vi "main - 截取字符显示.vi"() -> ()   [LabVIEW 2018]
uses:
  <vilib>/Instr/_visa.llb/VISA Configure Serial Port (Instr).vi
panel:
  out "波形图表 2":u32(graph)
  out "*(类型 *) &x 2":u32
  out "波形图表":u32(graph)
  out "Serial flag":bool
  out "*(类型 *) &x":u32
  out "子字符串 3":string
  out "子字符串 2":string
  out "子字符串":string
  out "枚举":T1
  out "返回数":u32
  in  "baud rate":u64(ring) items=["9600"=9600, "14400"=14400, "115200"=115200]
  out "read buffer":string
  out "serial_state":bool
  in  "serial":refnum<visa-resource-name> caption="serial_select"
  in  "serial_open":bool
  in  "exit":bool
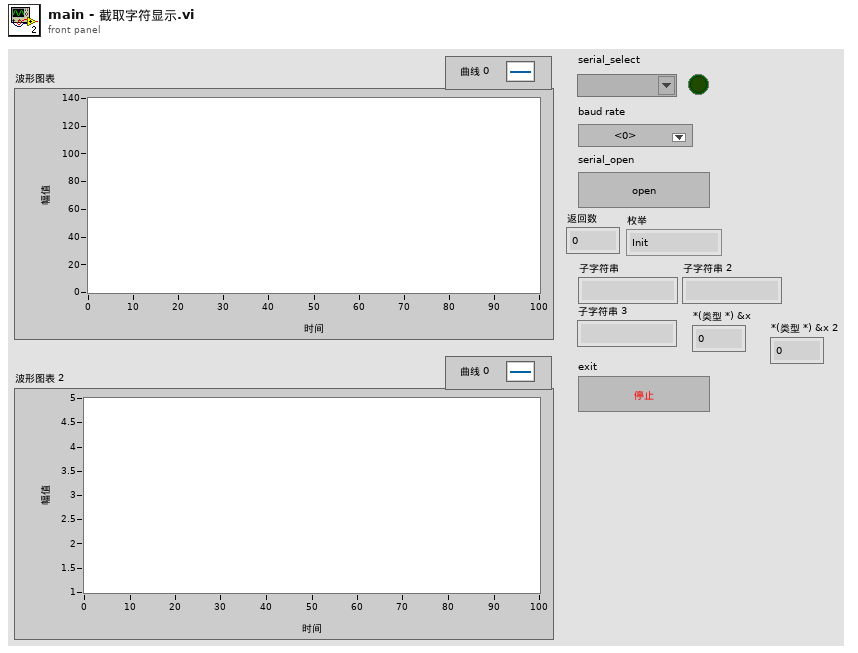
[diagram p1: front panel]
types:
  T1 = typedef "状态机.ctl" = enum16{"Init", "Send", "Wait", "GetData", "Deal", "Exit"}
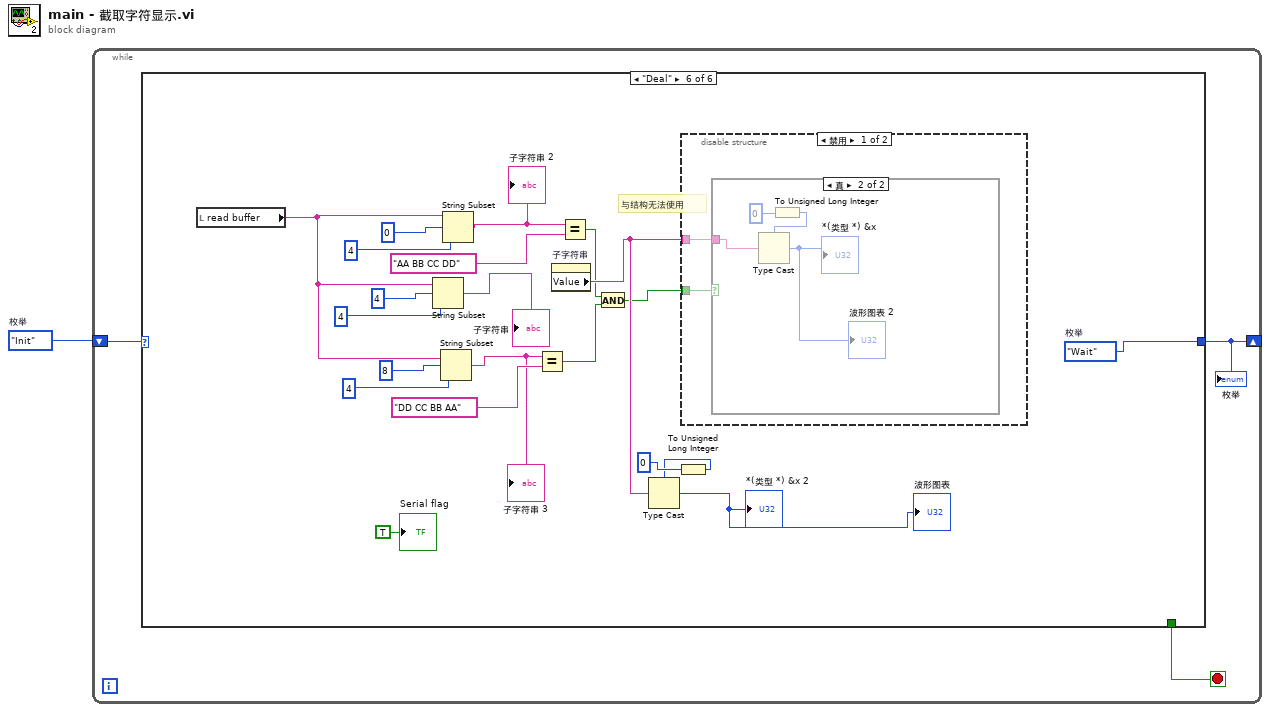
[diagram p0: block diagram]
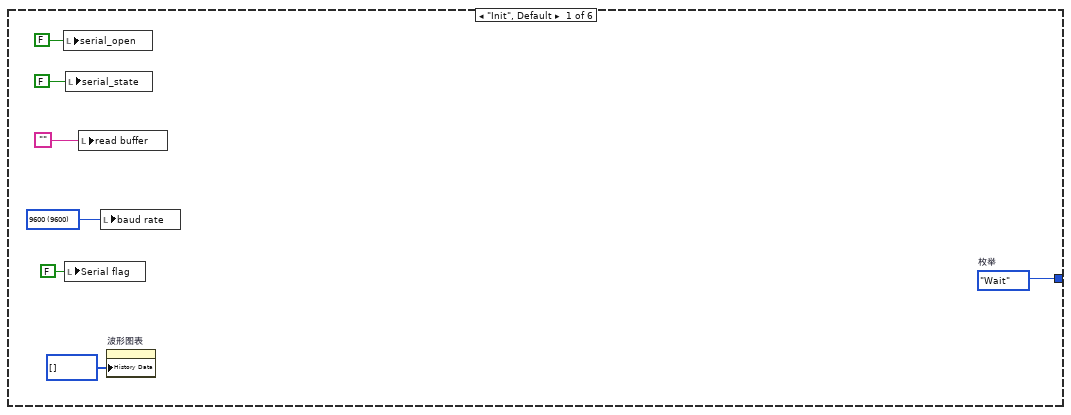
[diagram p2: hidden frame]
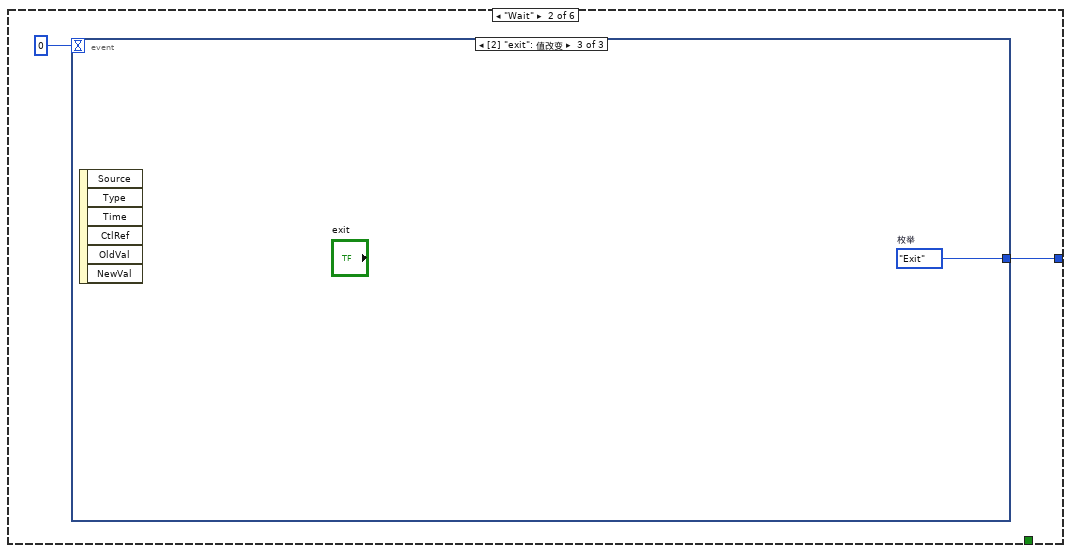
[diagram p3: hidden frame]
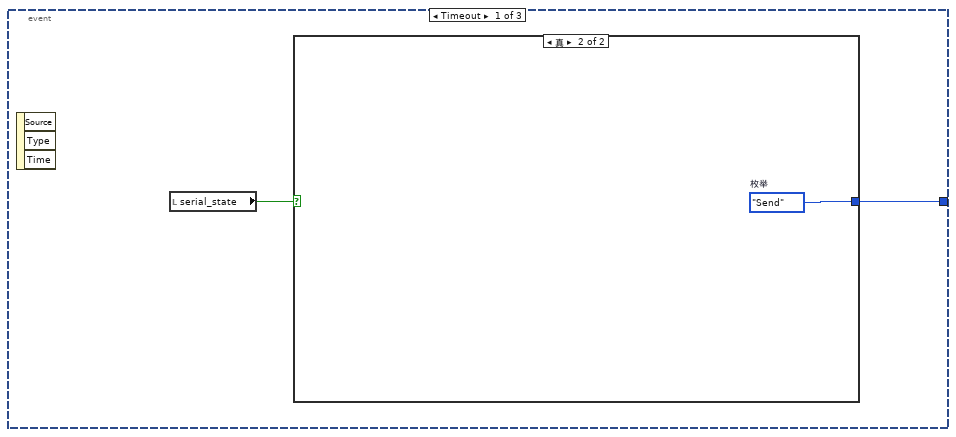
[diagram p4: hidden frame]
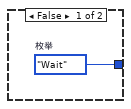
[diagram p5: hidden frame]
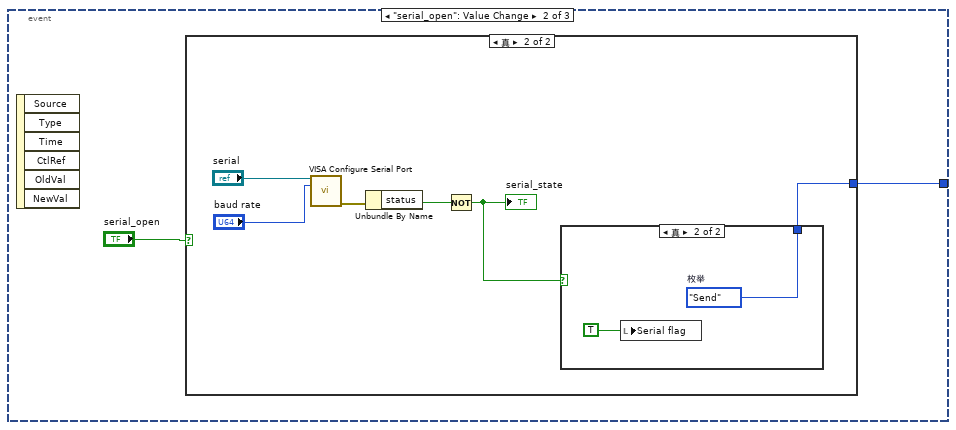
[diagram p6: hidden frame]
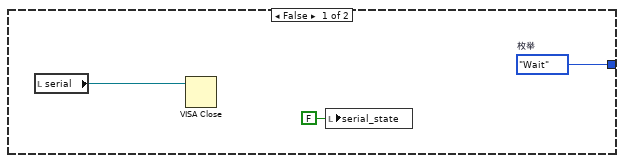
[diagram p7: hidden frame]
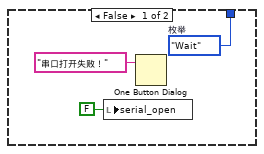
[diagram p8: hidden frame]
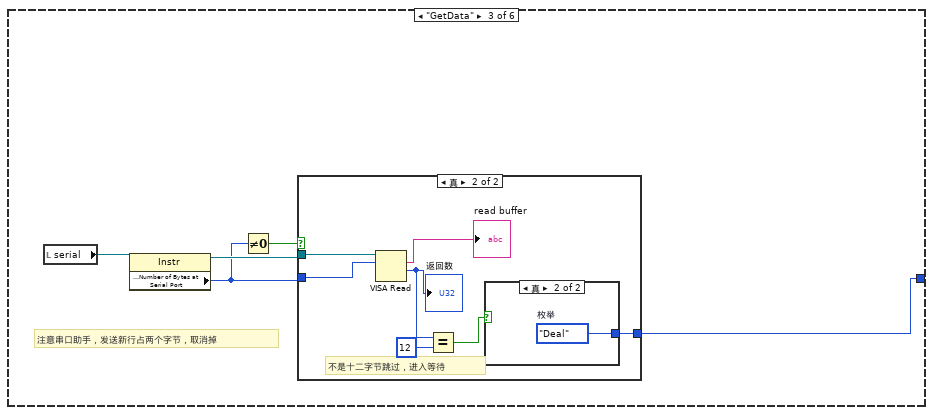
[diagram p9: hidden frame]
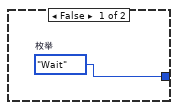
[diagram p10: hidden frame]
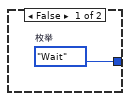
[diagram p11: hidden frame]
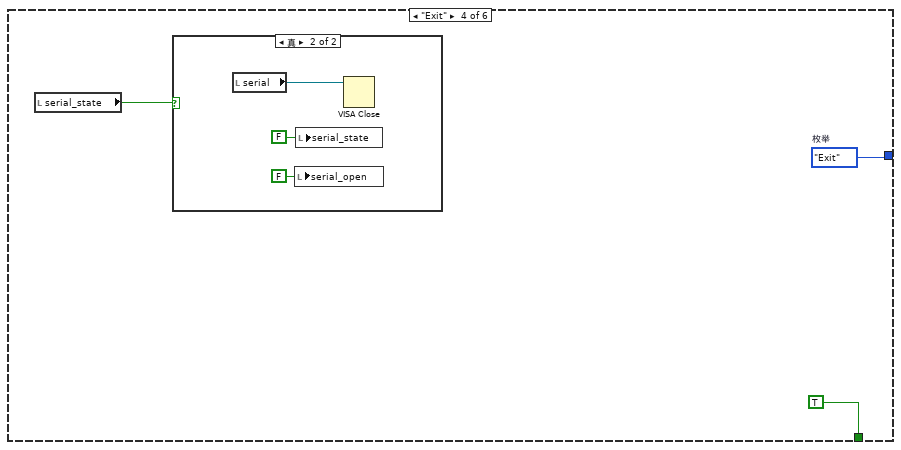
[diagram p12: hidden frame]
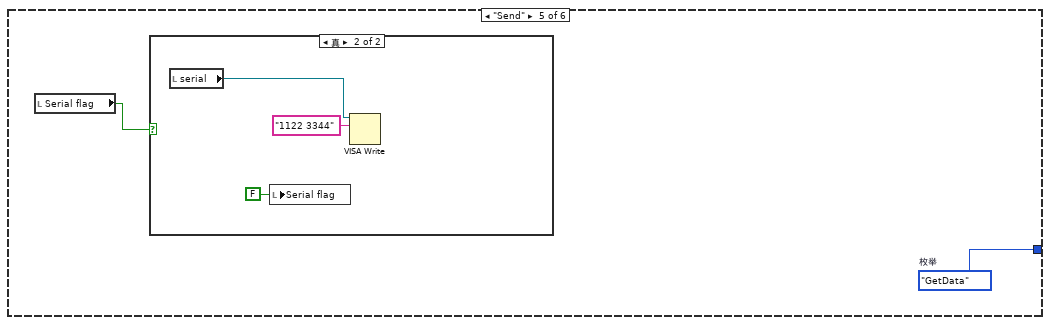
[diagram p14: hidden frame]
diagram:
  w1 = 状态机."Init"  # 枚举
  n1 = while {
    shift-right: [w3] -> _
    shift-left: w1 -> [w4]
    stop <- w2 stop-if-true
    n2 = case shown="\"Deal\"" w4 {
      tunnel: [w9 w12 w35 w52 w56 w81] -> w3
      tunnel: [_ _ _ TRUE _ _] -> w2
      frame "Init", Default {
        w7 = u64 9600 items=["9600"=9600, "115200"=115200] ("baud rate")
        w9 = 状态机."Wait"  # 枚举
        n3 = local write "serial_open"(FALSE ("serial_open")) -> ()
        n4 = local write "Serial flag"(FALSE ("Serial flag")) -> ()
        n5 = local write "serial_state"(FALSE ("serial_state")) -> ()
        n6 = local write "read buffer"("") -> ()
        n7 = local write "baud rate"(w7) -> ()
        n8 = property on="波形图表" class="WFChart (严格)"("History Data"=u32[] [] ("历史数据")) -> ()  [unwired: 2 in, 2 out]
      }
      frame "Wait" {
        n9 = event shown="[2] \"exit\": 值改变" {
          selector: _ -> [_ _ _]
          dyn-events: _ -> [_ _ _]
          timeout: 0 -> [_ _ _]
          tunnel: [w14 w18 w34] -> w12
          event Timeout {
            n10 = event-data() -> ()  [unwired: 1 in, 3 out]
            n11 = local read "serial_state"() -> (w15:bool)
            n12 = case shown="真" w15 {
              tunnel: [w16 w17] -> w14
              frame False {
                w16 = 状态机."Wait"  # 枚举
              }
              frame True {
                w17 = 状态机."Send"  # 枚举
              }
            }
          }
          event "serial_open": Value Change {
            n13 = event-data() -> ()  [unwired: 1 in, 6 out]
            n14 = case shown="真" "serial_open" {
              tunnel: [w20 w24] -> w18
              frame False {
                w20 = 状态机."Wait"  # 枚举
                n15 = local read "serial"() -> (w22:refnum<visa-resource-name>)
                n16 = VISA Close(VISA resource name=w22) -> ()  [unwired: 1 in, 1 out]
                n17 = local write "serial_state"(FALSE ("serial_state")) -> ()
              }
              frame True {
                n18 = call-poly "VISA Configure Serial Port"("VISA resource name"="serial", "baud rate (9600)"="baud rate") -> ("error out"=w27:errorcluster)  [unwired: 12 in, 1 out]
                n19 = Unbundle By Name(w27) -> ("status"=w26:bool)
                n20 = Not(x=w26) -> (.not. x?=w25:bool)
                "serial_state" <- w25
                n21 = case shown="真" w25 {
                  tunnel: [w29 w33] -> w24
                  frame False {
                    w29 = 状态机."Wait"  # 枚举
                    n22 = local write "serial_open"(FALSE ("serial_open")) -> ()
                    n23 = One Button Dialog(message="串口打开失败！" ("消息")) -> ()  [unwired: 1 in, 1 out]
                  }
                  frame True {
                    w33 = 状态机."Send"  # 枚举
                    n24 = local write "Serial flag"(TRUE ("Serial flag")) -> ()
                  }
                }
              }
            }
          }
          event "exit": Value Change {
            w34 = 状态机."Exit"  # 枚举
            n25 = event-data() -> ()  [unwired: 1 in, 6 out]
          }
        }
      }
      frame "GetData" {
        # "注意串口助手，发送新行占两个字节，取消掉"
        n26 = local read "serial"() -> (w36:refnum<visa-resource-name>)
        n27 = property class="Instr"(reference=w36) -> (reference out=w39:refnum<visa-resource-name>, "Serial Settings:Number of Bytes at Serial Port"=w37:u32)  [unwired: 1 in, 1 out]
        n28 = Not Equal To 0?(x=w37) -> (x != 0?=w38:bool)
        n29 = case shown="真" w38 {
          tunnel: w39 -> [_ w47]
          tunnel: w37 -> [_ w46]
          tunnel: [w40 w41] -> w35
          frame False {
            w40 = 状态机."Wait"  # 枚举
          }
          frame True {
            # "不是十二字节跳过，进入等待"
            n30 = VISA Read(VISA resource name=w47, byte count=w46) -> (read buffer=→"read buffer":string, return count=w44:u32)  [unwired: 1 in, 2 out]
            "返回数" <- w44
            n31 = Equal?(x=w44, y=u32 12) -> (x = y?=w42:bool)
            n32 = case shown="真" w42 {
              tunnel: [w48 w49] -> w41
              frame False {
                w48 = 状态机."Wait"  # 枚举
              }
              frame True {
                w49 = 状态机."Deal"  # 枚举
              }
            }
          }
        }
      }
      frame "Exit" {
        w52 = 状态机."Exit"  # 枚举
        n33 = local read "serial_state"() -> (w50:bool)
        n34 = case shown="真" w50 {
          frame False {
          }
          frame True {
            n35 = local read "serial"() -> (w55:refnum<visa-resource-name>)
            n36 = local write "serial_open"(FALSE ("serial_state")) -> ()
            n37 = local write "serial_state"(FALSE ("serial_state")) -> ()
            n38 = VISA Close(VISA resource name=w55) -> ()  [unwired: 1 in, 1 out]
          }
        }
      }
      frame "Send" {
        w56 = 状态机."GetData"  # 枚举
        n39 = local read "Serial flag"() -> (w57:bool)
        n40 = case shown="真" w57 {
          frame False {
          }
          frame True {
            n41 = local read "serial"() -> (w59:refnum<visa-resource-name>)
            n42 = local write "Serial flag"(FALSE ("Serial flag")) -> ()
            n43 = VISA Write(VISA resource name=w59, write buffer="1122 3344" ("写入缓冲区")) -> ()  [unwired: 1 in, 3 out]
          }
        }
      }
      frame "Deal" {
        w81 = 状态机."Wait"  # 枚举
        # "与结构无法使用"
        n44 = local read "read buffer"() -> (w74:string)
        n45 = String Subset(string=w74, offset (0)=4 ("偏移量(0)"), length (rest)=4 ("长度（剩余）")) -> (substring=→"子字符串":string)
        n46 = String Subset(string=w74, offset (0)=8 ("偏移量(0)"), length (rest)=4 ("长度（剩余）")) -> (substring=w63:string)
        "子字符串 3" <- w63
        n47 = String Subset(string=w74, offset (0)=0 ("偏移量(0)"), length (rest)=4 ("长度（剩余）")) -> (substring=w62:string)
        "子字符串 2" <- w62
        n48 = Equal?(x=w63, y="DD CC BB AA") -> (x = y?=w61:bool)
        n49 = property on="子字符串" class="Str"() -> ("Value"=w68:string)  [unwired: 2 in, 2 out]
        n50 = Equal?(x=w62, y="AA BB CC DD") -> (x = y?=w64:bool)
        n51 = And(x=w64, y=w61) -> (x .and. y?=w65:bool)
        n52 = To Unsigned Long Integer(number=0) -> (unsigned 32bit integer=w69:u32)
        n53 = Type Cast(type=w69, x=w68) -> (*(type *) &x=→"波形图表" →"*(类型 *) &x 2":u32)
        n54 = disable-structure shown="禁用" {
          disable-tunnel: w68 -> [w83 _]
          disable-tunnel: w65 -> [w82 _]
          frame Disabled {
            n55 = case shown="真" w82 {
              tunnel: w83 -> [_ w87]
              frame False {
              }
              frame True {
                n56 = To Unsigned Long Integer(number=0) -> (unsigned 32bit integer=w85:u32)
                n57 = Type Cast(type=w85, x=w87) -> (*(type *) &x=→"*(类型 *) &x" →"波形图表 2":u32)
              }
            }
          }
          frame Enabled {
          }
        }
        "Serial flag" <- TRUE ("Serial flag")
      }
    }
    "枚举" <- w3
  }
